vi "VerifGuider.vi"(8 "error in (no error)":errorcluster, 11 "S4GUI in":refnum<class "S4GUI.lvclass">) -> (0 "error out":errorcluster, 3 "S4GUI out":refnum<class "S4GUI.lvclass">)   [LabVIEW 2018, in "S4GUI.lvclass"]
uses:
  S4GUI.lvclass
  S4GUI.lvclass/S4GUI.ctl
  GSserver/GSserver.lvclass
  GSstatus/GSstatus.lvclass
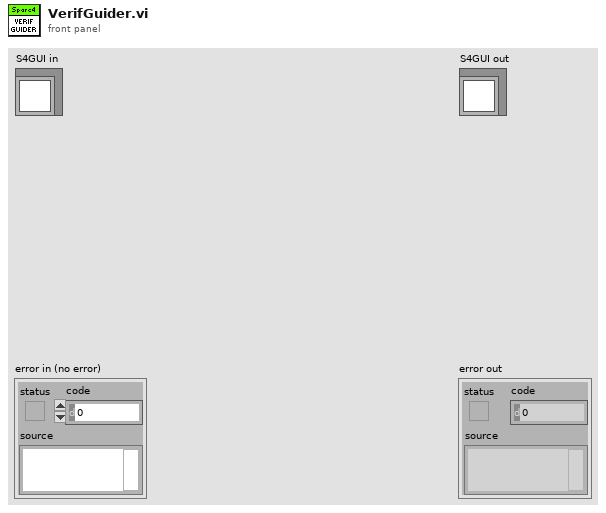
[diagram p1: front panel]
types:
  T1 = cluster{"FocusPhot":dbl, "FocusPolar":dbl, "FocusEffic":dbl, "FocusInstrum":dbl, "ICS":bool, "AG":bool, "BROKER":string, "timestamp":string, "FocusPos":dbl, "MirrorPos":dbl}
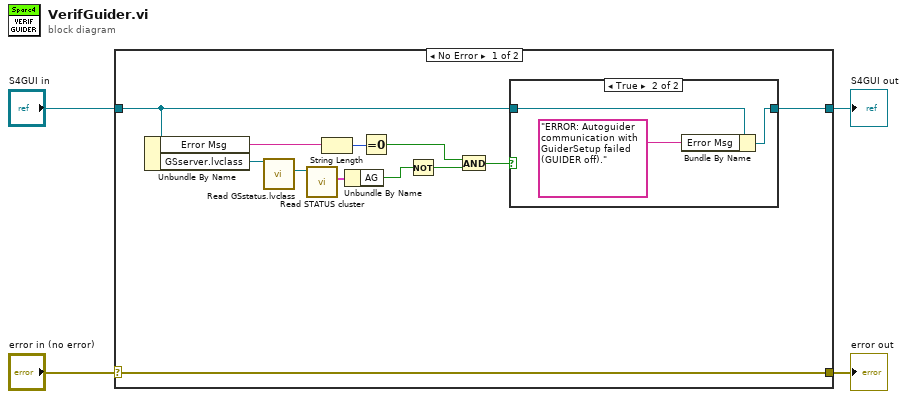
[diagram p0: block diagram]
diagram:
  n1 = case shown="No Error" "error in (no error)" {
    selector: "error in (no error)" -> [w16 w22]
    tunnel: [w16 w22] -> w3
    tunnel: [w10 w21] -> w1
    tunnel: "S4GUI in" -> [w11 w21]
    frame No Error {
      n2 = Unbundle By Name(w11) -> ("Error Msg"=w13:string, "GSserver.lvclass"=w15:refnum<class "GSserver.lvclass">)
      n3 = call-dynamic "Read GSstatus.lvclass.vi"("GSserver in"=w15) -> ("GSstatus.lvclass"=w14:refnum<class "GSstatus.lvclass">)  [unwired: 8 in, 2 out]
      n4 = call-dynamic "Read STATUS cluster.vi"("GSstatus in"=w14) -> ("STATUS cluster"=w12:T1)  [unwired: 8 in, 2 out]
      n5 = String Length(string=w13) -> (length=w9:i32)
      n6 = Unbundle By Name(w12) -> ("AG"=w7:bool)
      n7 = Equal To 0?(x=w9) -> (x = 0?=w8:bool)
      n8 = Not(x=w7) -> (.not. x?=w5:bool)
      n9 = And(x=w8, y=w5) -> (x .and. y?=w6:bool)
      n10 = case shown="True" w6 {
        tunnel: [w17 w19] -> w10
        tunnel: w11 -> [w17 w20]
        frame False {
        }
        frame True {
          n11 = Bundle By Name(cluster=w20, "Error Msg"="ERROR: Autoguider communication with GuiderSetup failed (GUIDER off).") -> (w19:refnum<class "S4GUI.lvclass">)
        }
      }
    }
    frame Error {
    }
  }
  "error out" <- w3
  "S4GUI out" <- w1
